vi "Begin.vi"(8 "error in":errorcluster) -> (0 "error out":errorcluster)   [LabVIEW 2014]
doc: "Called before other user functions, this VI is expected to open initial I/O refnums, load in file data, and do all program initialization. Notice that the <B>error out</B> terminal is simply used for data flow. Wiring it to other structures or subVIs ensures that this VI runs first."
uses:
  <vilib>/Rock Robotics/WPI/SafetyOutput/WPI_SafetyOutputConfigMenu.ctl
  <vilib>/Rock Robotics/WPI/DriverStation/WPI_DriverStationRobotMode2.ctl
  <vilib>/Rock Robotics/WPI/Joystick/WPI_JoystickDeviceEnum.ctl
  <vilib>/Rock Robotics/SystemInterfaces/DIO/FPGA_DIOPWMChannel.ctl
  <vilib>/Rock Robotics/WPI/Solenoid/WPI_SolenoidChannel.ctl
  <vilib>/Rock Robotics/SystemInterfaces/DIO/FPGA_DIOChannel.ctl
  <vilib>/Rock Robotics/SystemInterfaces/Typedef/FPGA_TypedefAnalogModule.ctl
  <vilib>/Rock Robotics/SystemInterfaces/AI/FPGA_AIChannel.ctl
  <vilib>/Rock Robotics/SystemInterfaces/Typedef/FPGA_TypedefDigitalModule.ctl
  Robot Global Data.vi
  <vilib>/Rock Robotics/Network Tables/SD Write String Array.vi
  <vilib>/Rock Robotics/WPI/RobotDrive/WPI_RobotDriveOpen4MotorWithTalon.vi
  <vilib>/Rock Robotics/WPI/MotorControl/WPI_MotorControlOpen Talon.vi
  <vilib>/Rock Robotics/WPI/RobotDrive/WPI_RobotDriveOpen2MotorWithTalon.vi
  <vilib>/Rock Robotics/WPI/Solenoid/WPI_SolenoidOpenSingle.vi
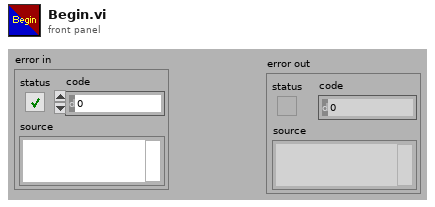
[diagram p1: front panel]
types:
  T1 = typedef "FPGA_DIOPWMChannel.ctl" = enum8{"PWM 0", "PWM 1", "PWM 2", "PWM 3", "PWM 4", "PWM 5", "PWM 6", "PWM 7", "PWM 8", "PWM 9", "PWM MXP 0", "PWM MXP 1", "PWM MXP 2", "PWM MXP 3", "PWM MXP 4", "PWM MXP 5", "PWM MXP 6", "PWM MXP 7", "PWM MXP 8", "PWM MXP 9", "Invalid"}
  T2 = typedef "FPGA_TypedefDigitalModule.ctl" = enum16{"Controller 1"}
  T3 = typedef "FPGA_AIChannel.ctl" = enum8{"AI 0", "AI 1", "AI 2", "AI 3", "AI MXP 0", "AI MXP 1", "AI MXP 2", "AI MXP 3", "Invalid"}
  T4 = typedef "FPGA_TypedefAnalogModule.ctl" = enum16{"Controller 1"}
  T5 = typedef "FPGA_DIOChannel.ctl" = enum8{"DIO 0", "DIO 1", "DIO 2", "DIO 3", "DIO 4", "DIO 5", "DIO 6", "DIO 7", "DIO 8", "DIO 9", "DIO MXP 0", "DIO MXP 1", "DIO MXP 2", "DIO MXP 3", "DIO MXP 4", "DIO MXP 5", "DIO MXP 6", "DIO MXP 7", "DIO MXP 8", "DIO MXP 9", "DIO MXP 10", "DIO MXP 11", "DIO MXP 12", "DIO MXP 13", "DIO MXP 14", "DIO MXP 15", "Invalid"}
  T6 = typedef "WPI_SolenoidChannel.ctl" = enum8{"Solenoid 0", "Solenoid 1", "Solenoid 2", "Solenoid 3", "Solenoid 4", "Solenoid 5", "Solenoid 6", "Solenoid 7", "Invalid"}
  T7 = typedef "WPI_JoystickDeviceEnum.ctl" = enum16{"USB 0", "USB 1", "USB 2", "USB 3", "USB 4", "USB 5"}
  T8 = typedef "WPI_DriverStationRobotMode2.ctl" = enum16{"Autonomous Disabled", "Autonomous Enabled", "Teleop Disabled", "Teleop Enabled", "Disconnected", "Finish", "Test Disabled", "Test Enabled", "Emergency Stopped"}
  T9 = typedef "WPI_SafetyOutputConfigMenu.ctl" = enum16{"Enable", "Disable"}
  T10 = typedef "WPI_DigitalInputDevRef.ctl" = cluster{"DevStatus":errorcluster, "DIO Channel":T5, "Controller":T2}
  T11 = typedef "WPI_ServoDeviceRef.ctl" = cluster{"DeviceStatus":errorcluster, "Controller":T2, "PWM Channel":T1, "DeadBand":T12}
  T12 = typedef "WPI_PWMDeadband.ctl" = cluster{"Name":string, "maxPositivePwm":i32, "minPositivePwm":i32, "centerPwm":i32, "maxNegativePwm":i32, "minNegativePwm":i32, "angularRange":u16}
  T13 = typedef "WPI_AnalogChannelDevRef.ctl" = cluster{"DevStatus":errorcluster, "Controller":T4, "Analog Channel":T3}
  T14 = typedef "WPI_RobotDriveDevRef.ctl" = cluster{"DevStatus":errorcluster, "Motors[]":T15[], "Square Inputs":bool, "Max Output":dbl}
  T15 = typedef "WPI_MotorControlDeviceRef.ctl" = cluster{"DeviceStatus":errorcluster, "Type":T16, "PWM":cluster{"Controller":T2, "PWM Channel":T1, "DeadBand":T12}, "CAN":cluster{"Device Number":u8, "Control Mode":T17, "Semaphore":T18, "Max Vout":dbl, "TalonSRX Control Mode":T19}, "Invert":bool, "TransformRef":T20, "InvTransformRef":T20}
  T16 = typedef "WPI_MotorControlType.ctl" = enum16{"PWM", "CAN", "CANTalonSRX"}
  T17 = typedef "WPI_CANJaguar_ControlMode.ctl" = enum8{"Percent VBus", "Current", "Speed", "Position", "Voltage"}
  T18 = typedef "Semaphore RefNum" = refnum<k1>
  T19 = typedef "WPI_CANTalonSRX_APIControlMode.ctl" = enum8{"Percent VBus", "Speed", "Position", "Slave", "Unchanged / Invalid"}
  T20 = typedef "WPI_PWMTransform_ConPane.ctl" = refnum<vi>
  T21 = typedef "WPI_JoystickDevRef.ctl" = cluster{"Device":T7}
  T22 = typedef "WPI_SolenoidDevRef.ctl" = cluster{"DevStatus":errorcluster, "Pneumatics Control Module":u8, "Forward Solenoid Channel":T6, "Reverse Solenoid Channel":T6}
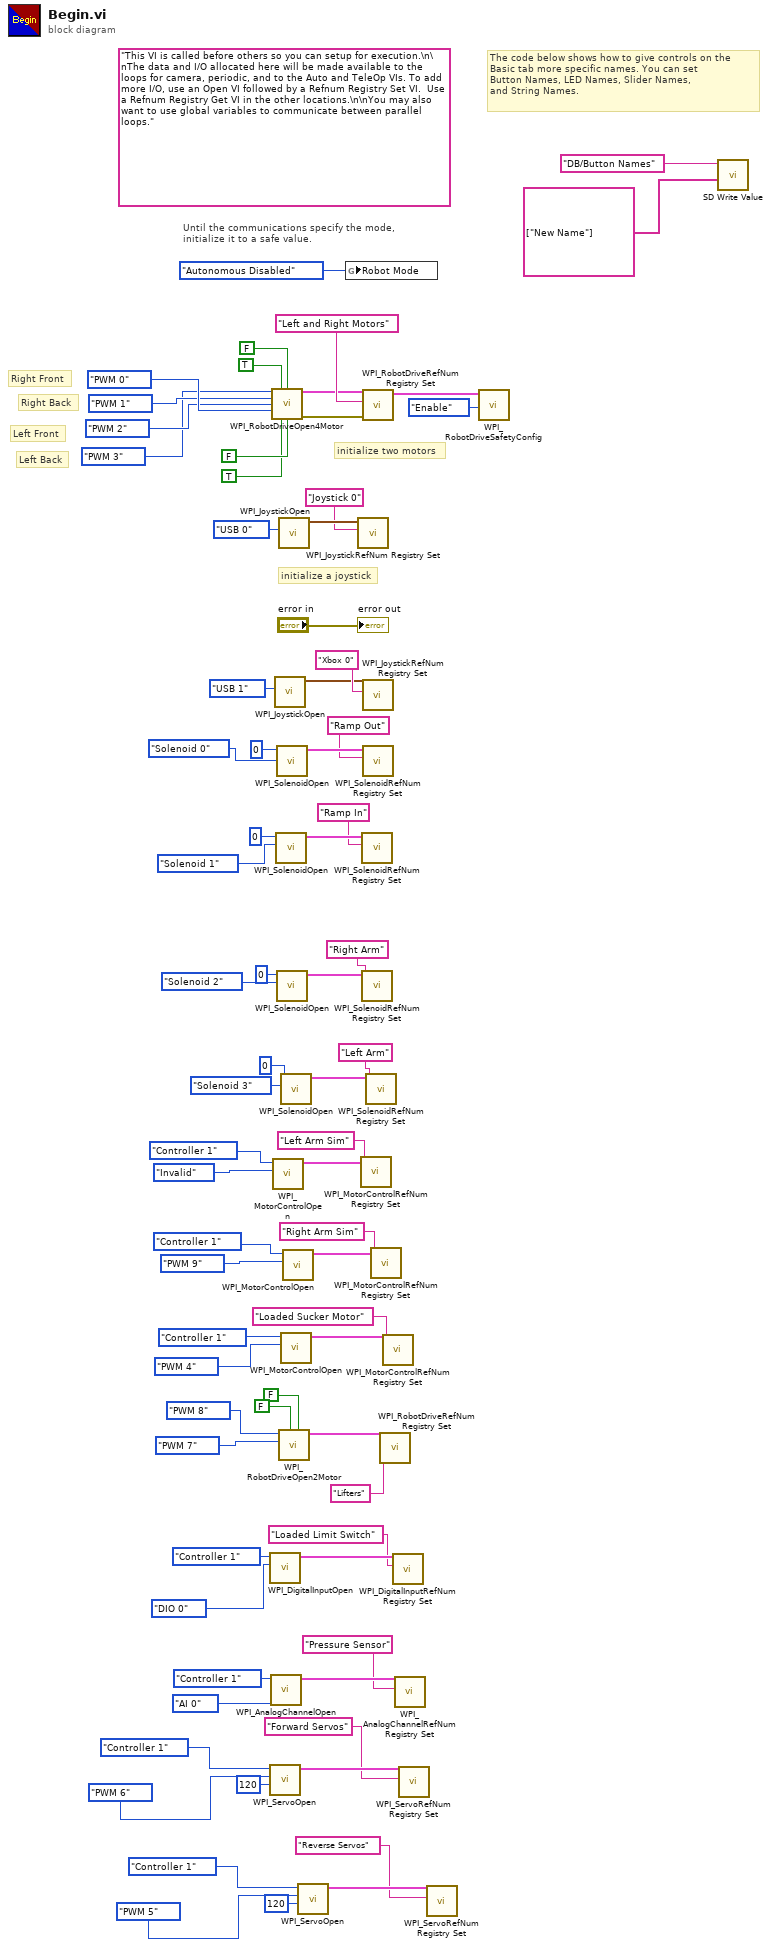
[diagram p0: block diagram]
diagram:
  (unwired) "This VI is called before others so you can setup for execution.\n\nThe data and I/O allocated here will be made available to the loops for camera, periodic, and to the Auto and TeleOp VIs. To add more I/O, use an Open VI followed by a Refnum Registry Set VI.  Use a Refnum Registry Get VI in the other locations.\n\nYou may also want to use global variables to communicate between parallel loops."
  # "Left Back"
  # "Left Front"
  # "Right Back"
  # "Right Front"
  # "The code below shows how to give controls on the\nBasic tab more specific names. You can set\nButton Names, LED Names, Slider Names,\nand String Names."
  # "initialize a joystick"
  # "Until the communications specify the mode,\ninitialize it to a safe value."
  # "initialize two motors"
  n1 = call <vilib>:"WPI_DigitalInputOpen.vi"("DIO Channel"=FPGA_DIOChannel."DIO 0", "Controller"=FPGA_TypedefDigitalModule."Controller 1") -> ("DigitalInputDevRef"=w23:T10)  [unwired: 8 in, 1 out]
  n2 = call <vilib>:"WPI_ServoOpen.vi"("Angular Range"=u16 120, "PWM Channel"=FPGA_DIOPWMChannel."PWM 6", "Controller"=FPGA_TypedefDigitalModule."Controller 1") -> ("ServoDeviceRef"=w10:T11)  [unwired: 7 in, 1 out]
  n3 = call <vilib>:"WPI_AnalogChannelOpen.vi"("Analog Channel"=FPGA_AIChannel."AI 0", "Controller"=FPGA_TypedefAnalogModule."Controller 1") -> ("AIDeviceRef"=w16:T13)  [unwired: 8 in, 1 out]
  n4 = call-poly <vilib>:"WPI_RobotDriveOpen4Motor.vi"("Rear Left Motor"=FPGA_DIOPWMChannel."PWM 3", "Rear Left Motor Inverted"=TRUE, "Rear Right Motor Inverted"=FALSE, "Rear Right Motor"=FPGA_DIOPWMChannel."PWM 1", "Front Left Motor"=FPGA_DIOPWMChannel."PWM 2", "Front Right Motor"=FPGA_DIOPWMChannel."PWM 0", "Front Left Motor Inverted"=TRUE, "Front Right Motor Inverted"=FALSE) -> ("RobotDriveDevRef"=w63:T14, "error out"=w62:errorcluster)  [unwired: 6 in]
  n5 = call-poly <vilib>:"WPI_MotorControlOpen.vi"("PWM Channel"=FPGA_DIOPWMChannel."Invalid", "Controller"=FPGA_TypedefDigitalModule."Controller 1") -> ("MotorControlDeviceRef"=w43:T15)  [unwired: 8 in, 1 out]
  n6 = call <vilib>:"WPI_JoystickOpen.vi"("JoystickDevice"=WPI_JoystickDeviceEnum."USB 1") -> ("JoystickDevRef"=w64:T21)  [unwired: 10 in]
  n7 = call-poly <vilib>:"WPI_SolenoidOpen.vi"("Solenoid Channel"=WPI_SolenoidChannel."Solenoid 1" ("Reverse Solenoid Channel"), "Pneumatics Control Module (0)"=u8 0) -> ("SolenoidDevRef"=w14:T22)  [unwired: 8 in, 1 out]
  n8 = call-poly <vilib>:"WPI_SolenoidOpen.vi"("Solenoid Channel"=WPI_SolenoidChannel."Solenoid 0" ("Forward Solenoid Channel"), "Pneumatics Control Module (0)"=u8 0) -> ("SolenoidDevRef"=w52:T22)  [unwired: 8 in, 1 out]
  n9 = call-poly <vilib>:"WPI_SolenoidOpen.vi"("Solenoid Channel"=WPI_SolenoidChannel."Solenoid 2", "Pneumatics Control Module (0)"=u8 0) -> ("SolenoidDevRef"=w51:T22)  [unwired: 8 in, 1 out]
  n10 = call <vilib>:"WPI_JoystickOpen.vi"("JoystickDevice"=WPI_JoystickDeviceEnum."USB 0") -> ("JoystickDevRef"=w71:T21)  [unwired: 10 in]
  n11 = call-poly <vilib>:"WPI_RobotDriveOpen2Motor.vi"("Right Motor Inverted"=FALSE, "Left Motor Inverted"=FALSE, "Right Motor"=FPGA_DIOPWMChannel."PWM 7", "Left Motor"=FPGA_DIOPWMChannel."PWM 8") -> ("RobotDriveDevRef"=w35:T14)  [unwired: 6 in, 1 out]
  n12 = call-poly <vilib>:"WPI_SolenoidOpen.vi"("Solenoid Channel"=WPI_SolenoidChannel."Solenoid 3", "Pneumatics Control Module (0)"=u8 0) -> ("SolenoidDevRef"=w48:T22)  [unwired: 8 in, 1 out]
  n13 = call-poly <vilib>:"WPI_MotorControlOpen.vi"("PWM Channel"=FPGA_DIOPWMChannel."PWM 4", "Controller"=FPGA_TypedefDigitalModule."Controller 1") -> ("MotorControlDeviceRef"=w27:T15)  [unwired: 8 in, 1 out]
  n14 = call-poly <vilib>:"WPI_MotorControlOpen.vi"("PWM Channel"=FPGA_DIOPWMChannel."PWM 9", "Controller"=FPGA_TypedefDigitalModule."Controller 1") -> ("MotorControlDeviceRef"=w39:T15)  [unwired: 8 in, 1 out]
  n15 = call <vilib>:"WPI_ServoOpen.vi"("Angular Range"=u16 120, "PWM Channel"=FPGA_DIOPWMChannel."PWM 5", "Controller"=FPGA_TypedefDigitalModule."Controller 1") -> ("ServoDeviceRef"=w5:T11)  [unwired: 7 in, 1 out]
  n16 = global write "Robot Global Data.vi" "Robot Mode"(WPI_DriverStationRobotMode2."Autonomous Disabled" ("Robot Mode")) -> ()
  n17 = call <vilib>:"WPI_JoystickRefNum Registry Set.vi"("refnum name"="Joystick 0", "JoystickDevRef"=w71) -> ()  [unwired: 8 in, 2 out]
  n18 = call <vilib>:"WPI_MotorControlRefNum Registry Set.vi"("refnum name"="Left Arm Sim", "MotorControlDevRef"=w43) -> ()  [unwired: 8 in, 2 out]
  n19 = call <vilib>:"WPI_SolenoidRefNum Registry Set.vi"("refnum name"="Ramp In", "SolenoidDevRef"=w14) -> ()  [unwired: 8 in, 2 out]
  n20 = call <vilib>:"WPI_SolenoidRefNum Registry Set.vi"("refnum name"="Right Arm", "SolenoidDevRef"=w51) -> ()  [unwired: 8 in, 2 out]
  n21 = call <vilib>:"WPI_RobotDriveRefNum Registry Set.vi"("error in (no error)"=w62, "refnum name"="Left and Right Motors", "RobotDriveDevRef"=w63) -> ("RobotDriveDevRef"=w74:T14)  [unwired: 8 out]
  n22 = call <vilib>:"WPI_JoystickRefNum Registry Set.vi"("refnum name"="Xbox 0", "JoystickDevRef"=w64) -> ()  [unwired: 8 in, 2 out]
  n23 = call <vilib>:"WPI_SolenoidRefNum Registry Set.vi"("refnum name"="Ramp Out", "SolenoidDevRef"=w52) -> ()  [unwired: 8 in, 2 out]
  n24 = call <vilib>:"WPI_SolenoidRefNum Registry Set.vi"("refnum name"="Left Arm", "SolenoidDevRef"=w48) -> ()  [unwired: 8 in, 2 out]
  n25 = call <vilib>:"WPI_MotorControlRefNum Registry Set.vi"("refnum name"="Right Arm Sim", "MotorControlDevRef"=w39) -> ()  [unwired: 8 in, 2 out]
  n26 = call <vilib>:"WPI_RobotDriveRefNum Registry Set.vi"("refnum name"="Lifters", "RobotDriveDevRef"=w35) -> ()  [unwired: 8 in, 2 out]
  n27 = call <vilib>:"WPI_MotorControlRefNum Registry Set.vi"("refnum name"="Loaded Sucker Motor", "MotorControlDevRef"=w27) -> ()  [unwired: 8 in, 2 out]
  n28 = call <vilib>:"WPI_DigitalInputRefNum Registry Set.vi"("refnum name"="Loaded Limit Switch", "DigitalInputDevRef"=w23) -> ()  [unwired: 8 in, 2 out]
  n29 = call <vilib>:"WPI_AnalogChannelRefNum Registry Set.vi"("refnum name"="Pressure Sensor", "AIDeviceRef"=w16) -> ()  [unwired: 8 in, 2 out]
  n30 = call <vilib>:"WPI_ServoRefNum Registry Set.vi"("refnum name"="Forward Servos", "ServoDeviceRef"=w10) -> ()  [unwired: 8 in, 2 out]
  n31 = call <vilib>:"WPI_ServoRefNum Registry Set.vi"("refnum name"="Reverse Servos", "ServoDeviceRef"=w5) -> ()  [unwired: 8 in, 2 out]
  n32 = call <vilib>:"WPI_RobotDriveSafetyConfig.vi"("mode"=WPI_SafetyOutputConfigMenu."Enable", "RobotDriveDevRef"=w74) -> ()  [unwired: 8 in, 2 out]
  n33 = call-poly <vilib>:"SD Write Value.vi"("String Array"=string[] ["New Name"], "Name"="DB/Button Names") -> ()  [unwired: 8 in, 2 out]
  "error out" <- "error in"
